vi "connect.vi"(3 "error in":errorcluster, 4 "Simulator Port":i32, 5 "Simulator IP":string) -> (0 "error out":errorcluster, 2 "TCP Network Connection Out":refnum<k5>)   [LabVIEW 2019]
doc: "Open a TCP connection given an IP and control port."
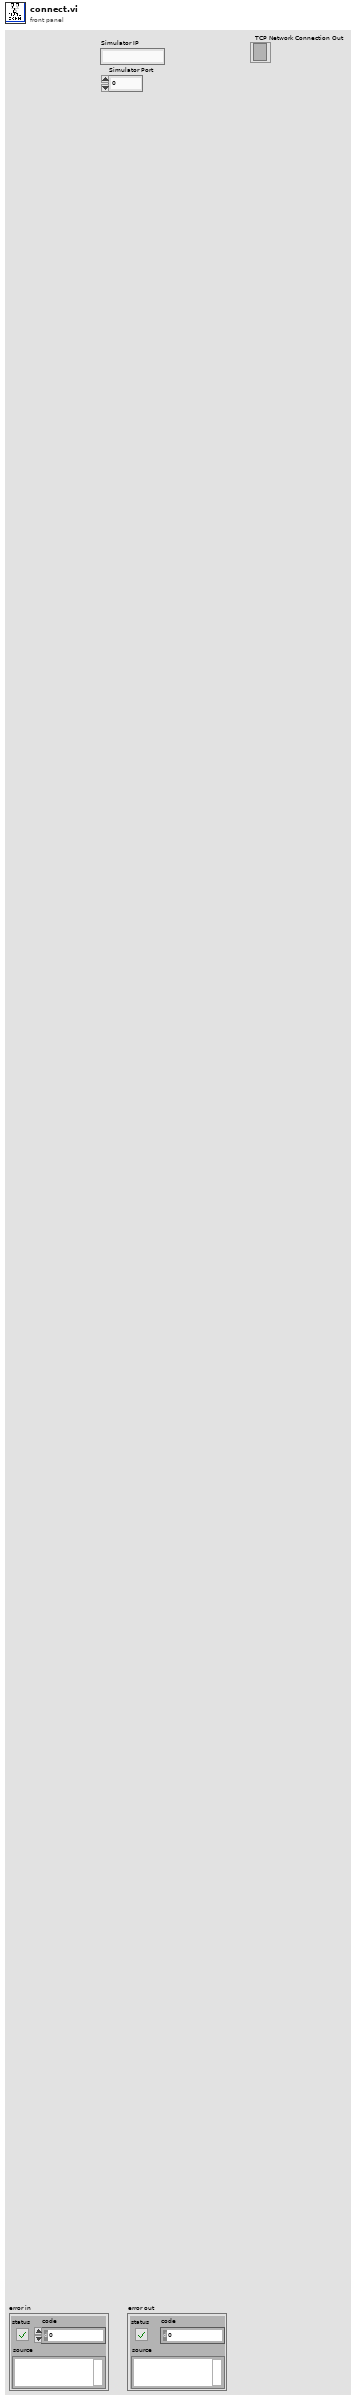
[diagram p1: front panel]
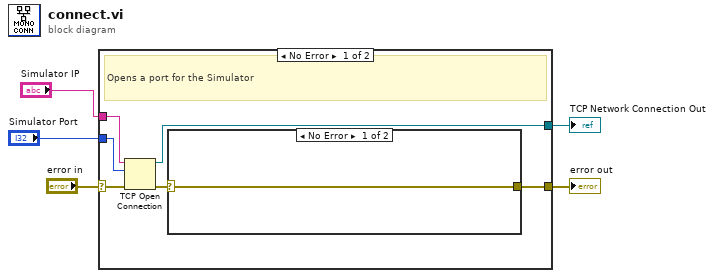
[diagram p0: block diagram]
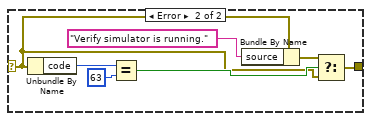
[diagram p2: hidden frame]
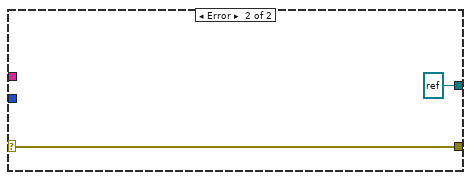
[diagram p3: hidden frame]
diagram:
  n1 = case shown="No Error" "error in" {
    selector: "error in" -> [w9 w21]
    tunnel: [w6 w21] -> w5
    tunnel: [w7 refnum<k5> refnum ("connection ID")] -> w4
    tunnel: "Simulator IP" -> [w11 _]
    tunnel: "Simulator Port" -> [w10 _]
    frame No Error {
      # "Opens a port for the Simulator"
      n2 = TCP Open Connection(address=w11, remote port or service name=w10, error in (no error)=w9) -> (connection ID=w7:refnum<k5>, error out=w8:errorcluster)  [unwired: 2 in]
      n3 = case shown="No Error" w8 {
        selector: w8 -> [w12 w14]
        tunnel: [w12 w13] -> w6
        frame No Error {
        }
        frame Error {
          n4 = Unbundle By Name(w14) -> ("code"=w19:i32)
          n5 = Equal?(x=w19, y=63) -> (x = y?=w16:bool)
          n6 = Bundle By Name(cluster=w14, "source"="Verify simulator is running.") -> (w15:errorcluster)
          n7 = Select(t=w15, s=w16, f=w14) -> (s? t:f=w13:errorcluster)
        }
      }
    }
    frame Error {
    }
  }
  "error out" <- w5
  "TCP Network Connection Out" <- w4
